vi "S2C_Shared_Func_Response.vi"(8 "Error In":errorcluster, 9 "Timeout":dbl, 10 "Func-Q":refnum<queue>, 11 "Command":string) -> (0 "Error Out":errorcluster, 3 "Response":string)   [LabVIEW 2015]
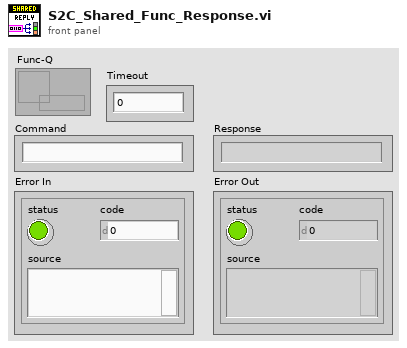
[diagram p1: front panel]
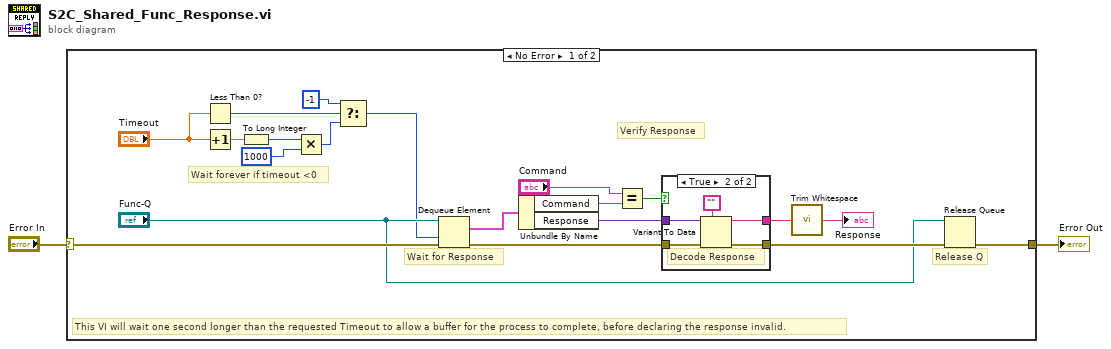
[diagram p0: block diagram]
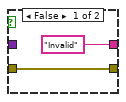
[diagram p2: hidden frame]
diagram:
  n1 = case shown="No Error" "Error In" {
    selector: "Error In" -> [w12 w30]
    tunnel: [w13 w30] -> w1
    frame No Error {
      # "This VI will wait one second longer than the requested Timeout to allow a buffer for the process to complete, before declaring the response invalid."
      # "Wait forever if timeout <0"
      # "Release Q"
      # "Verify Response"
      # "Wait for Response"
      n2 = Less Than 0?(x="Timeout") -> (x < 0?=w7:bool)
      n3 = Increment(x="Timeout") -> (x+1=w16:dbl)
      n4 = To Long Integer(number=w16) -> (32bit integer=w15:i32)
      n5 = Multiply(x=w15, y=1000) -> (x*y=w6:i32)
      n6 = Select(t=-1, s=w7, f=w6) -> (s? t:f=w4:i32)
      n7 = Dequeue Element(queue="Func-Q", timeout in ms (-1)=w4, error in (no error)=w12) -> (element=w21:cluster{"Command":string, "Response":variant}, error out=w22:errorcluster)  [unwired: 2 out]
      n8 = Unbundle By Name(w21) -> ("Command"=w19:string, "Response"=w20:variant)
      n9 = Equal?(x="Command", y=w19) -> (x = y?=w18:bool)
      n10 = case shown="True" w18 {
        tunnel: w22 -> [w24 w29]
        tunnel: w20 -> [_ w28]
        tunnel: [w24 w27] -> w17
        tunnel: ["Invalid" w25] -> w9
        frame False {
        }
        frame True {
          # "Decode Response"
          n11 = Variant To Data(error in=w29, type="", Variant=w28) -> (data=w25:string, error out=w27:errorcluster)
        }
      }
      n12 = call <vilib>:"Trim Whitespace.vi"("string"=w9) -> ("trimmed string"=→"Response":string)  [unwired: 1 in]
      n13 = Release Queue(queue="Func-Q", error in (no error)=w17) -> (error out=w13:errorcluster)  [unwired: 1 in, 2 out]
    }
    frame Error {
    }
  }
  "Error Out" <- w1
